vi "Flip (Greyscale).vi"(7 "Flip Mode (Default: X-Axis)":T1, 8 "error in (no error)":errorcluster, 10 "Greyscale Destination Image":T2, 11 "Greyscale Source Image":T2) -> (0 "error out":errorcluster, 3 "Greyscale Destination Image (duplicate)":T2)   [LabVIEW 2020, in "g_ar_toolkit.image.lvlib"]
uses:
  g_ar_toolkit.image.lvlib
  Greyscale Image.ctl
  Flip Mode.ctl
  348de330-10c9-445f-8d54-7780e9118077.vi
  g_ar_toolkit.common/Module Path.vi
  <vilib>/Utility/error.llb/Error Cluster From Error Code.vi
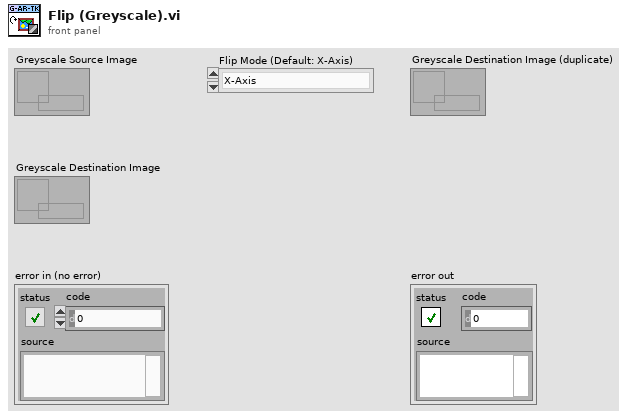
[diagram p1: front panel]
types:
  T1 = typedef "g_ar_toolkit.image.lvlib/Flip Mode.ctl" = enum8{"X-Axis", "Y-Axis", "X and Y Axes"}
  T2 = typedef "g_ar_toolkit.image.lvlib/Greyscale Image.ctl" = refnum<data-value>
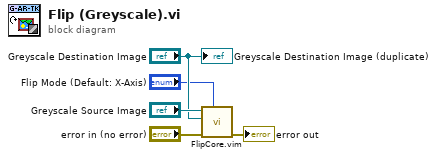
[diagram p0: block diagram]
diagram:
  n1 = call "FlipCore.vim"("Flip Mode"="Flip Mode (Default: X-Axis)", "error in (no error)"="error in (no error)", "Destination Image"="Greyscale Destination Image", "Source Image"="Greyscale Source Image") -> ("error out"=→"error out":errorcluster)  [unwired: 7 in]
  "Greyscale Destination Image (duplicate)" <- "Greyscale Destination Image"
